vi "Value to String.vi"(8 "error in (no error)":errorcluster, 11 "NT Enum in":refnum<class "NT Enum.lvclass">) -> (0 "error out":errorcluster, 2 "string":string, 3 "NT Enum out":refnum<class "NT Enum.lvclass">)   [LabVIEW 2020, in "PV Access.lvlib" / "PV Data.lvlib" / "NT Enum.lvclass"]
uses:
  NT Enum.lvclass
  NT Enum.lvclass/NT Enum.ctl
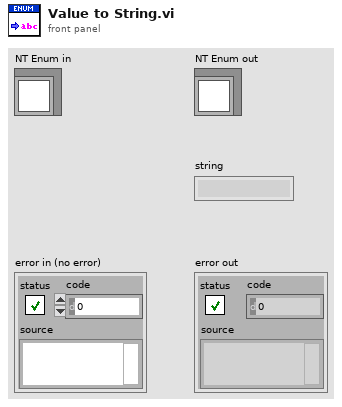
[diagram p1: front panel]
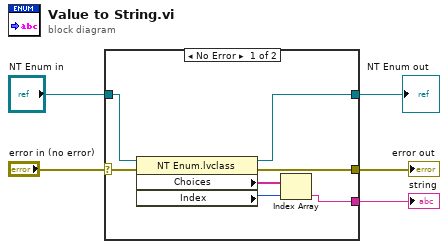
[diagram p0: block diagram]
diagram:
  n1 = case shown="No Error" "error in (no error)" {
    selector: "error in (no error)" -> [w12 w13]
    tunnel: [w11 w13] -> w4
    tunnel: [w6 w14] -> w2
    tunnel: "NT Enum in" -> [w10 w14]
    tunnel: [w7 _] -> w1
    frame No Error {
      n2 = property class="NT Enum.lvclass"(reference=w10, error in=w12) -> (reference out=w6:refnum<class "NT Enum.lvclass">, error out=w11:errorcluster, "Choices"=w9:string[], "Index"=w8:i32)
      n3 = Index Array(array=w9, index=w8) -> (element=w7:string)
    }
    frame Error {
    }
  }
  "error out" <- w4
  "NT Enum out" <- w2
  "string" <- w1
